vi "Teleop.vi"(10 "Match Info":T1={"Autonomous Elapsed Seconds"=0.0, "TeleOp Elapsed Seconds"=0.0, "Disabled Elapsed Seconds"=0.0, "Visited Autonomous"=FALSE, "Visited TeleOp"=FALSE, "Visited Disabled"=FALSE, "Autonomous Settings"={"Autonomous Style"=enum."Independent", "VI Refnum"=refnum}}, 11 "Call Context":T2) -> ()   [LabVIEW 2015]
doc: "This VI is called for each TeleOp packet received from the DS where the robot is not disabled. It is often used to read from the joysticks and update I/O or to update setpoints for timed control loops. It should complete and return within 20 milliseconds or it may miss DS packets."
uses:
  <vilib>/Rock Robotics/WPI/DriverStation/WPI_DriverStationDerivedRobotMode.ctl
  <vilib>/Rock Robotics/WPI/DriverStation/WPI_DriverStationMatch Info.ctl
  sprocket/src/Refname/Refname Enum (Joystick).ctl
  sprocket/src/Action/Action Name.ctl
  sprocket/src/Refname/Refname to String (Joystick).vi
  Robot Global Data.vi
  <vilib>/Rock Robotics/WPI/Joystick/WPI_JoystickGetSetRefNum.vi
  sprocket/src/Typedefs/Logitech Axis Mapping.ctl
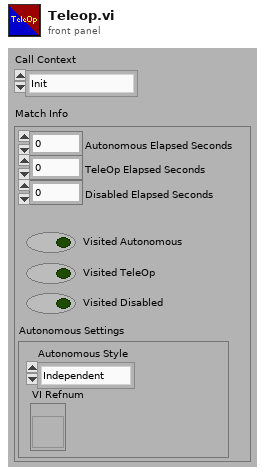
[diagram p1: front panel]
types:
  T1 = typedef "WPI_DriverStationMatch Info.ctl" = cluster{"Autonomous Elapsed Seconds":dbl, "TeleOp Elapsed Seconds":dbl, "Disabled Elapsed Seconds":dbl, "Visited Autonomous":bool, "Visited TeleOp":bool, "Visited Disabled":bool, "Autonomous Settings":cluster{"Autonomous Style":enum16{"Iterative", "Independent"}, "VI Refnum":refnum<vi>}}
  T2 = typedef "WPI_DriverStationDerivedRobotMode.ctl" = enum16{"Init", "Execute", "Stop"}
  T3 = typedef "Refname Enum (Joystick).ctl" = enum16{"Joystick 0", "Joystick 1", "Joystick 2", "Joystick 3"}
  T4 = typedef "WPI_JoystickDevRef.ctl" = cluster{"Device":T5}
  T5 = typedef "WPI_JoystickDeviceEnum.ctl" = enum16{"USB 0", "USB 1", "USB 2", "USB 3", "USB 4", "USB 5"}
  T6 = typedef "Logitech Axis Mapping.ctl" = enum32{"Left X Axis", "Left Y Axis", "Right X Axis", "Right Y Axis"}
  T7 = typedef "Action Name.ctl" = enum16{"No Action", "Drive Left", "Drive Right"}
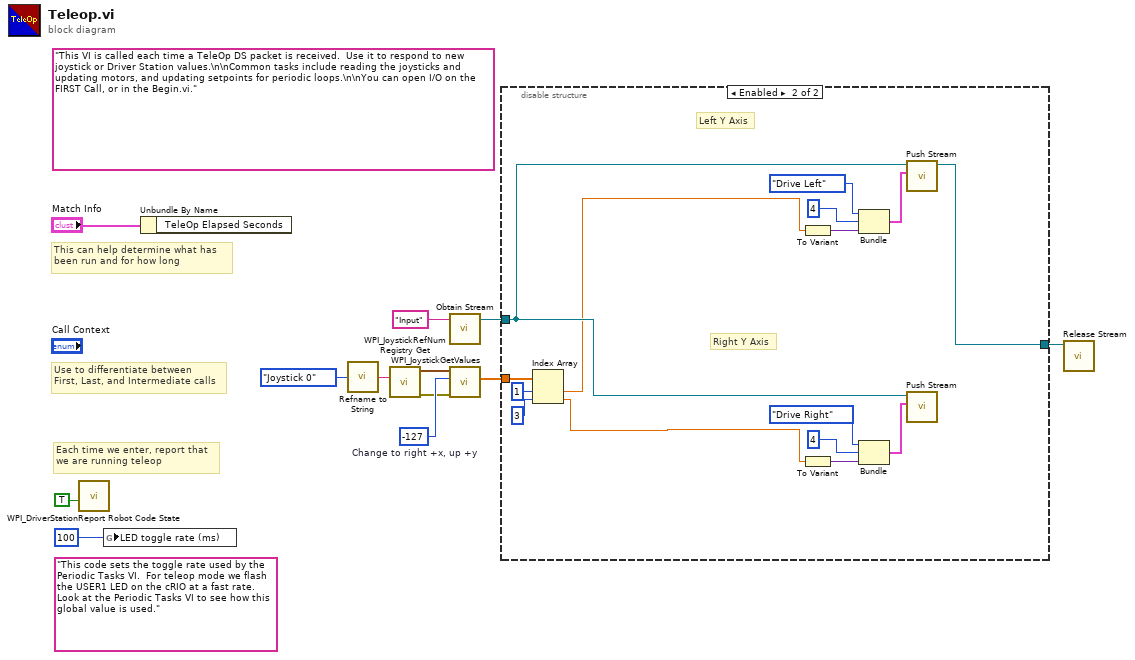
[diagram p0: block diagram]
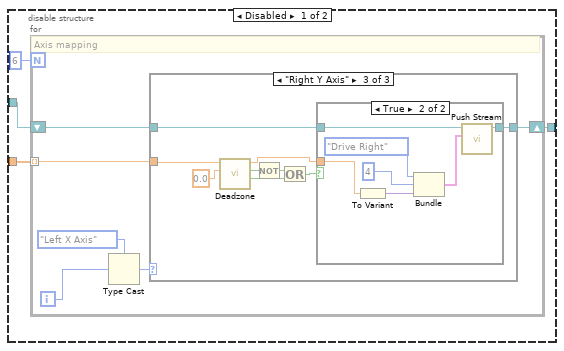
[diagram p2: hidden frame]
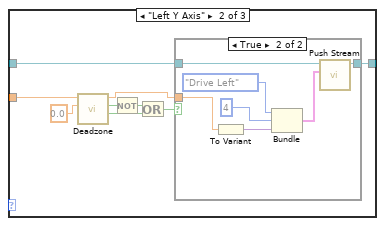
[diagram p4: hidden frame]
diagram:
  w6 = i8 -127  # Change to right +x, up +y
  (unwired) "This code sets the toggle rate used by the Periodic Tasks VI.  For teleop mode we flash the USER1 LED on the cRIO at a fast rate.  Look at the Periodic Tasks VI to see how this global value is used."
  (unwired) "This VI is called each time a TeleOp DS packet is received.  Use it to respond to new joystick or Driver Station values.\n\nCommon tasks include reading the joysticks and updating motors, and updating setpoints for periodic loops.\n\nYou can open I/O on the FIRST Call, or in the Begin.vi."
  # "Each time we enter, report that\nwe are running teleop"
  # "Use to differentiate between\nFirst, Last, and Intermediate calls"
  # "This can help determine what has\nbeen run and for how long"
  n1 = call <vilib>:"WPI_DriverStationReport Robot Code State.vi"("TeleOp"=TRUE ("Autonomous")) -> ()  [unwired: 10 in, 1 out]
  n2 = global write "Robot Global Data.vi" "LED toggle rate (ms)"(u32 100 ("LED ms toggle rate")) -> ()
  n3 = Unbundle By Name("Match Info") -> ()  [unwired: 1 out]
  n4 = call-poly "Refname to String.vi"("Joystick Refname"=Refname_Enum_(Joystick)."Joystick 0") -> ("Refnum Name"=w2:string)
  n5 = call <vilib>:"WPI_JoystickRefNum Registry Get.vi"("refnum name"=w2) -> ("error out"=w4:errorcluster, "JoystickDevRef"=w5:T4)  [unwired: 9 in]
  n6 = call "Obtain Stream.vi"("Name"="Input") -> ("stream out"=w8:refnum<queue>)  [unwired: 9 in, 1 out]
  n7 = call <vilib>:"WPI_JoystickGetValues.vi"("error in (no error)"=w4, "Scaler"=w6, "JoystickDevRef"=w5) -> ("Axes"=w7:dbl[])  [unwired: 4 in, 4 out]
  n8 = disable-structure shown="Enabled" {
    disable-tunnel: [w16 w72] -> w9
    disable-tunnel: w8 -> [w15 w71]
    disable-tunnel: w7 -> [w14 w70]
    frame Disabled {
      n9 = for {
        N: 6 -> [_]
        tunnel: w14 -> [w19] mode=indexing
        shift-right: [w17] -> w16
        shift-left: w15 -> [w18]
        i -> [w21]
        # "Axis mapping"
        n10 = Type Cast(type=Logitech_Axis_Mapping."Left X Axis" ("Axis Mapping"), x=w21) -> (*(type *) &x=w20:T6)
        n11 = case shown="\"Right Y Axis\"" w20 {
          tunnel: w19 -> [_ w28 w43]
          tunnel: w18 -> [w23 w25 w42]
          tunnel: [w23 w24 w41] -> w17
          frame Default {
          }
          frame "Left Y Axis" {
            n12 = call "Deadzone.vi"("Deadzone"=0.0, "Input"=w28) -> ("Just entered deadzone?"=w27:bool, "In deadzone?"=w31:bool, "Output"=w26:dbl)  [unwired: 6 in, 1 out]
            n13 = Not(x=w31) -> (.not. x?=w30:bool)
            n14 = Or(x=w30, y=w27) -> (x .or. y?=w32:bool)
            n15 = case shown="True" w32 {
              tunnel: w26 -> [_ w39]
              tunnel: w25 -> [w33 w35]
              tunnel: [w33 w34] -> w24
              frame False {
              }
              frame True {
                n16 = To Variant(anything=w39) -> (Variant=w40:variant)
                n17 = Bundle("Name"=Action_Name."Drive Left", 4, "Variant"=w40) -> (w36:cluster{"Name":T7, i32, "Variant":variant})  [unwired: 1 in]
                n18 = call "Push Stream.vi"("action"=w36, "stream in"=w35) -> ("stream out"=w34:refnum<queue>)  [unwired: 8 in, 1 out]
              }
            }
          }
          frame "Right Y Axis" {
            n19 = call "Deadzone.vi"("Deadzone"=0.0, "Input"=w43) -> ("Just entered deadzone?"=w45:bool, "In deadzone?"=w48:bool, "Output"=w44:dbl)  [unwired: 6 in, 1 out]
            n20 = Not(x=w48) -> (.not. x?=w47:bool)
            n21 = Or(x=w47, y=w45) -> (x .or. y?=w49:bool)
            n22 = case shown="True" w49 {
              tunnel: w44 -> [_ w56]
              tunnel: w42 -> [w50 w52]
              tunnel: [w50 w51] -> w41
              frame False {
              }
              frame True {
                n23 = To Variant(anything=w56) -> (Variant=w57:variant)
                n24 = Bundle("Name"=Action_Name."Drive Right", 4, "Variant"=w57) -> (w53:cluster{"Name":T7, i32, "Variant":variant})  [unwired: 1 in]
                n25 = call "Push Stream.vi"("action"=w53, "stream in"=w52) -> ("stream out"=w51:refnum<queue>)  [unwired: 8 in, 1 out]
              }
            }
          }
        }
      }
    }
    frame Enabled {
      # "Left Y Axis"
      # "Right Y Axis"
      n26 = Index Array(array=w70, index #1=1 ("index"), index #2=3 ("index")) -> (element #1=w58:dbl, element #2=w63:dbl)
      n27 = To Variant(anything=w58) -> (Variant=w62:variant)
      n28 = To Variant(anything=w63) -> (Variant=w67:variant)
      n29 = Bundle("Name"=Action_Name."Drive Left", 4, "Variant"=w62) -> (w59:cluster{"Name":T7, i32, "Variant":variant})  [unwired: 1 in]
      n30 = Bundle("Name"=Action_Name."Drive Right", 4, "Variant"=w67) -> (w64:cluster{"Name":T7, i32, "Variant":variant})  [unwired: 1 in]
      n31 = call "Push Stream.vi"("action"=w59, "stream in"=w71) -> ("stream out"=w72:refnum<queue>)  [unwired: 8 in, 1 out]
      n32 = call "Push Stream.vi"("action"=w64, "stream in"=w71) -> ()  [unwired: 8 in, 2 out]
    }
  }
  n33 = call "Release Stream.vi"("stream in"=w9) -> ()  [unwired: 9 in, 2 out]
